vi "test_Measurement_GetMetadata_ContainsExpectedMeasurementDetails.vi"(8 "error in":errorcluster) -> (0 "error out":errorcluster, 2 "result":string, 3 "pass":bool)   [LabVIEW 2021, in "MeasurementServerTests.lvlib" / "Measurement Service Tests.lvlib"]
uses:
  Measurement Service Tests.lvlib
  gRPC/Generated APIs/ni/measurementlink/measurement/v2/Measurement Service Client V2/RPC Messages/ni_measurementlink_measurement_v2_MeasurementDetails.ctl
  Continuous Counting Measurement2/Run Service.vi
  Continuous Counting Measurement/Run Non-reentrant Service.vi
  Continuous Counting Measurement2/Continuous Counting Measurement2.lvclass
  Continuous Counting Measurement/Continuous Counting Measurement.lvclass
  gRPC/Generated APIs/ni/measurementlink/measurement/v2/Measurement Service Client V2/Measurement Service Client V2.lvlib
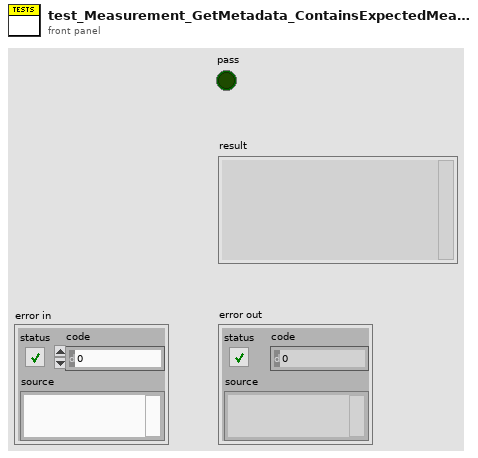
[diagram p1: front panel]
types:
  T1 = typedef "Measurement Service Client V2.lvlib/ni_measurementlink_measurement_v2_MeasurementDetails.ctl" = cluster{"display_name":string, "version":string}
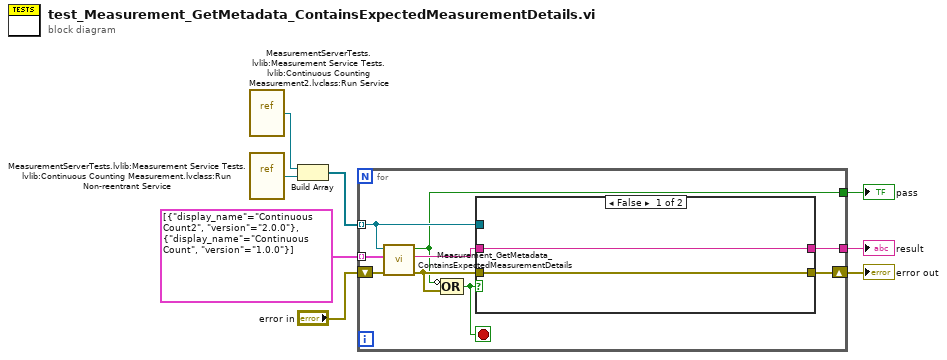
[diagram p0: block diagram]
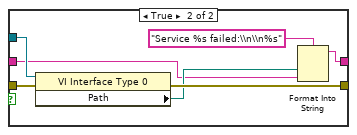
[diagram p2: hidden frame]
diagram:
  n1 = vi-ref "MeasurementServerTests.lvlib:Measurement Service Tests.lvlib:Continuous Counting Measurement2.lvclass:Run Service.vi"() -> (w4:refnum<vi>)
  n2 = vi-ref "MeasurementServerTests.lvlib:Measurement Service Tests.lvlib:Continuous Counting Measurement.lvclass:Run Non-reentrant Service.vi"() -> (w3:refnum<vi>)
  n3 = Build Array(w4, w3) -> (w2:refnum<vi>[])
  n4 = for {
    tunnel: [w16] -> w6
    tunnel: [w10] -> w5
    shift-right: [w15] -> w7
    shift-left: "error in" -> [w14]
    tunnel: w2 -> [w11] mode=indexing
    tunnel: T1[] [{"display_name"="Continuous Count2", "version"="2.0.0"}, {"display_name"="Continuous Count", "version"="1.0.0"}] ("expected measurement details") -> [w9] mode=indexing
    stop <- w17 stop-if-true
    n5 = call "Measurement_GetMetadata_ContainsExpectedMeasurementDetails.vi"("error in"=w14, "expected measurement details"=w9, "run service vi"=w11) -> ("error out"=w13:errorcluster, "result"=w12:string, "pass"=w10:bool)  [unwired: 6 in]
    n6 = Compound Arithmetic op=OR(invert w10, w13) -> (w17:bool)
    n7 = case shown="False" w17 {
      tunnel: w12 -> [w19 w21]
      tunnel: [w19 w20] -> w16
      tunnel: w11 -> [_ w26]
      tunnel: w13 -> [w18 w25]
      tunnel: [w18 w24] -> w15
      frame False {
      }
      frame True {
        n8 = property class="VI Interface Type 0"(reference=w26, error in=w25) -> (error out=w24:errorcluster, "Path"=w22:path)  [unwired: 1 out]
        n9 = Format Into String(format string="Service %s failed:\\n\\n%s", w22, w21) -> (resulting string=w20:string)  [unwired: 2 in, 1 out]
      }
    }
  }
  "pass" <- w5
  "result" <- w6
  "error out" <- w7
